vi "AlazarDSPGenerateWindowFunction.vi"(0 "Handle":u64, 1 "Window Type":u32(ring)=4 items=["None", "Hanning", "Hamming", "Blackman", "Blackman-Harris", "Bartlett"], 2 "window":sgl[](array[numeric]), 3 "WindowLength_samples":u32, 4 "PaddingLength_samples":u32, 5 "error in (no error)":errorcluster) -> (14 "Handle":u64, 15 "window":sgl[](array[numeric]), 18 "Return Code":u32, 19 "error out":errorcluster)   [LabVIEW 2009]
uses:
  ATSApi.dll
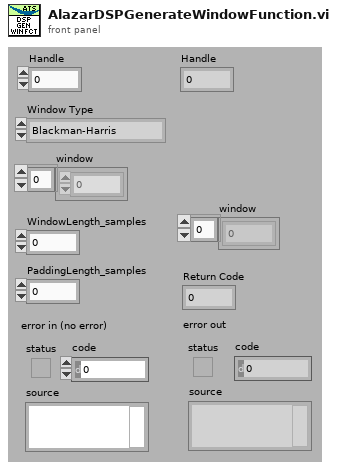
[diagram p1: front panel]
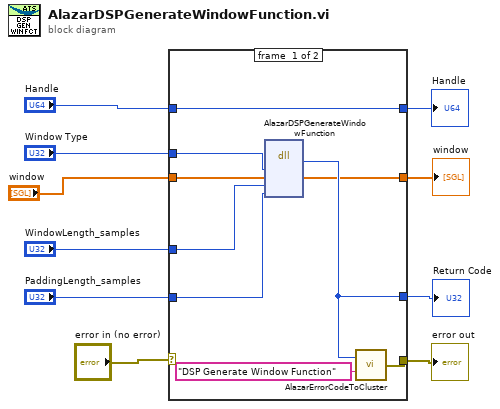
[diagram p0: block diagram]
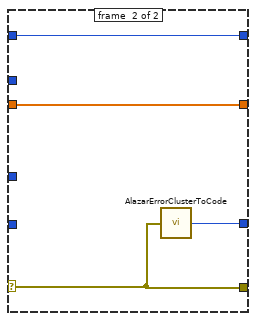
[diagram p2: hidden frame]
diagram:
  n1 = case shown="No Error" "error in (no error)" {
    selector: "error in (no error)" -> [_ w23]
    tunnel: [w17 w23] -> w9
    tunnel: [w19 w22] -> w8
    tunnel: "Handle" -> [w12 w21]
    tunnel: [w12 w21] -> w6
    tunnel: "window" -> [w16 w20]
    tunnel: "WindowLength_samples" -> [w15 _]
    tunnel: "PaddingLength_samples" -> [w14 _]
    tunnel: [w13 w20] -> w2
    tunnel: "Window Type" -> [w11 _]
    frame #0 {
      n2 = dll-call lib="ATSApi.dll" fn="AlazarDSPGenerateWindowFunction"("windowType"=w11, "window"=w16, "windowLength_samples"=w15, "paddingLength_samples"=w14) -> ("return type"=w19:u32, "window"=w13:sgl[])  [unwired: 6 in, 2 out]
      n3 = call "AlazarErrorCodeToCluster.vi"("Message"="DSP Generate Window Function", "Error Code"=w19) -> ("error out"=w17:errorcluster)
    }
    frame #1 {
      n4 = call "AlazarErrorClusterToCode.vi"("error in (no error)"=w23) -> ("Error Code"=w22:u32)
    }
  }
  "Handle" <- w6
  "error out" <- w9
  "Return Code" <- w8
  "window" <- w2
